vi "Firmware.vi"() -> ()   [LabVIEW 2025]
panel:
  in  "Stop Button":bool
  out "Progreso":u8(slide) scale=0.0..100.0
  out "Compilado":bool
  out "Subido":bool
  out "error_up":i32
  out "error_comp":i32
  in  "Upload Firmware":bool
  out "Lista de COMs":string[](array[string])
  out "error out":errorcluster
  in  "Selector":string(combo)
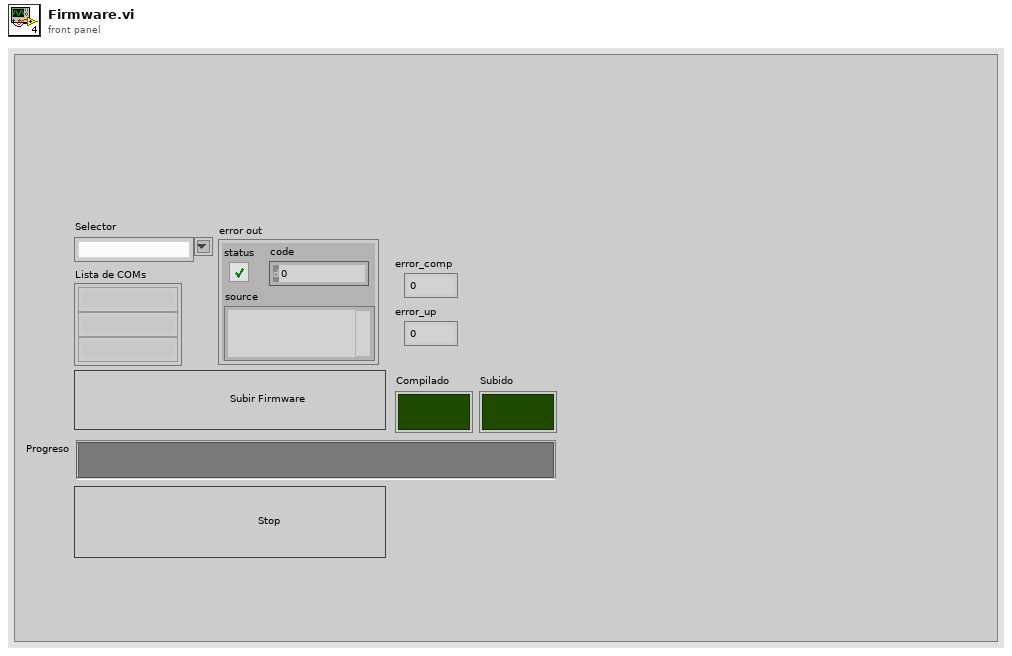
[diagram p1: front panel]
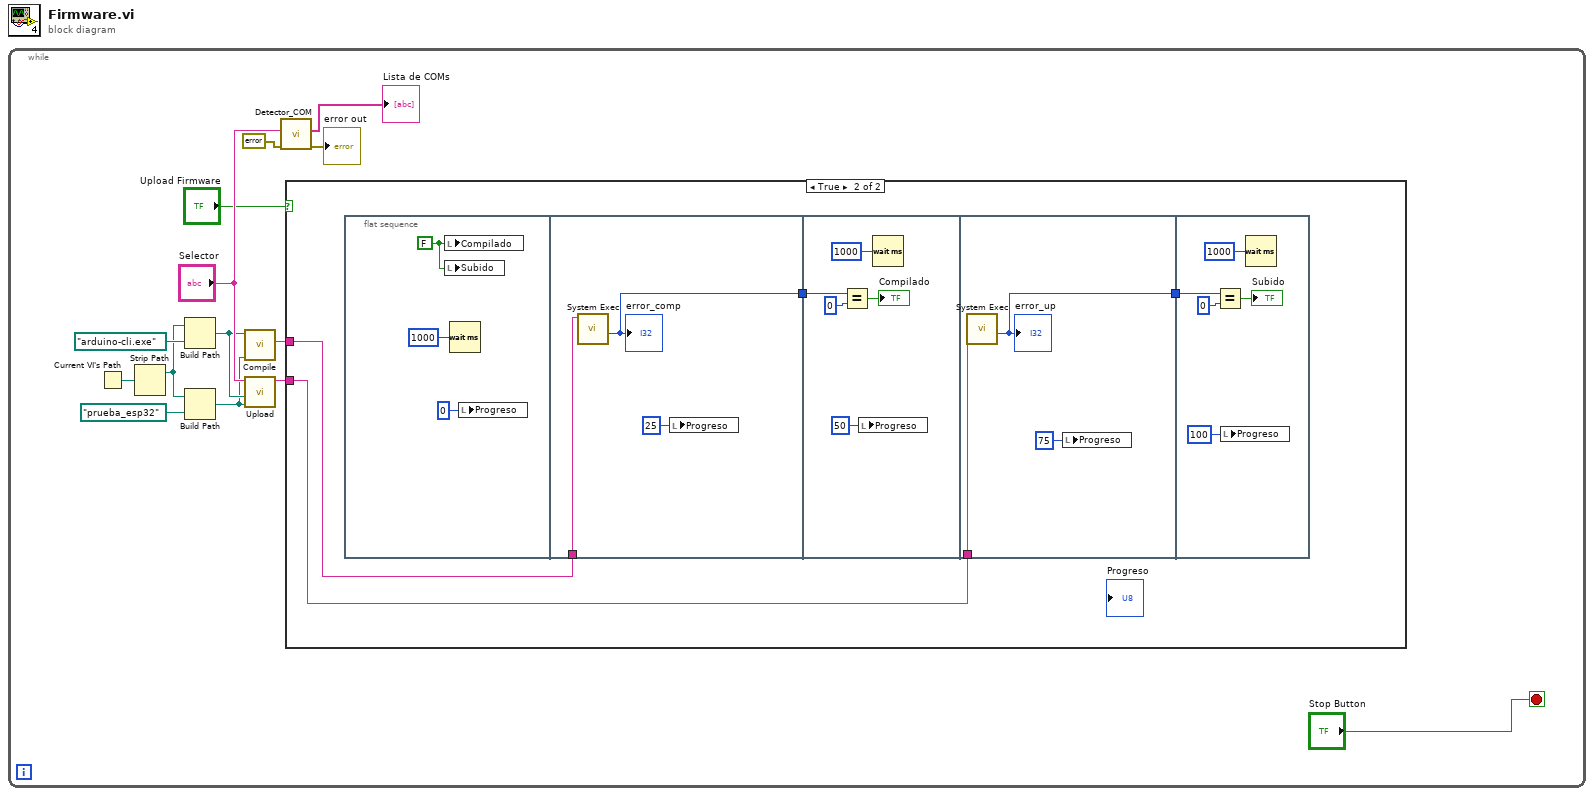
[diagram p0: block diagram]
diagram:
  n1 = while {
    stop <- "Stop Button" stop-if-true
    n2 = Current VI's Path() -> (path=w11:path)
    n3 = Strip Path(path=w11) -> (stripped path=w8:path)  [unwired: 1 out]
    n4 = Build Path(base path=w8, name or relative path=path "arduino-cli.exe") -> (appended path=w7:path)
    n5 = Build Path(base path=w8, name or relative path=path "prueba_esp32") -> (appended path=w6:path)
    n6 = call "Compile.vi"("INO"=w6, "CLI"=w7) -> ("concatenated string"=w3:string)  [unwired: 9 in]
    n7 = call "Upload.vi"("INO"=w6, "CLI"=w7, "Selector"="Selector") -> ("concatenated string"=w2:string)  [unwired: 8 in]
    n8 = call "Detector_COM.vi"("error in (no error)"=errorcluster {"status"=FALSE, "code"=0, "source"=""}, "Selector"="Selector") -> ("error out"=→"error out":errorcluster, "find list"=→"Lista de COMs":string[])  [unwired: 8 in]
    n9 = case shown="True" "Upload Firmware" {
      tunnel: w3 -> [_ w16]
      tunnel: w2 -> [_ w15]
      frame False {
      }
      frame True {
        n10 = flat-sequence {
          tunnel: [w24] -> w17
          tunnel: w16 -> [w23]
          tunnel: w17 -> [w27]
          tunnel: w15 -> [w32]
          tunnel: [w31] -> w18
          tunnel: w18 -> [w37]
          frame #0 {
            w21 = FALSE
            n11 = local write "Compilado"(w21) -> ()
            n12 = local write "Subido"(w21) -> ()
            n13 = Wait (ms)(milliseconds to wait=u32 1000) -> ()  [unwired: 1 out]
            n14 = local write "Progreso"(u8 0 ("Progreso")) -> ()
          }
          frame #1 {
            n15 = call <vilib>:"System Exec.vi"("command line"=w23) -> ("return code"=w24:i32)  [unwired: 7 in, 3 out]
            "error_comp" <- w24
            n16 = local write "Progreso"(u8 25 ("Progreso")) -> ()
          }
          frame #2 {
            n17 = Equal?(x=w27, y=0) -> (x = y?=→"Compilado":bool)
            n18 = local write "Progreso"(u8 50 ("Progreso")) -> ()
            n19 = Wait (ms)(milliseconds to wait=u32 1000) -> ()  [unwired: 1 out]
          }
          frame #3 {
            n20 = call <vilib>:"System Exec.vi"("command line"=w32) -> ("return code"=w31:i32)  [unwired: 7 in, 3 out]
            "error_up" <- w31
            n21 = local write "Progreso"(u8 75 ("Progreso")) -> ()
          }
          frame #4 {
            n22 = Equal?(x=w37, y=0) -> (x = y?=→"Subido":bool)
            n23 = local write "Progreso"(u8 100 ("Progreso")) -> ()
            n24 = Wait (ms)(milliseconds to wait=u32 1000) -> ()  [unwired: 1 out]
          }
        }
      }
    }
  }
